vi "Flush Written TDMS Data.vi"() -> ()   [LabVIEW 2023]
doc: "Demonstrates the use of the TDMS Flush function to flush any written data from memory to the .tdms file on disk."
uses:
  <vilib>/Utility/TDMS File Viewer/NI_TDMS File Viewer.lvlib
panel:
  in  "Stop":bool
  out "Graph":waveform(dbl)[](graph)
  # "Overview: Demonstrates the use of the TDMS Flush function to flush any written data from memory to the .tdms file on disk.\nInstructions:\n1. Run this VI.\n2. Click the Stop button to stop this VI and view the data written to the .tdms file.\n3. Open the block diagram of this example to understand how to use the TDMS Flush function to ensure data integrity.\n4. Delete the .tdms file (located at [LabVIEW Data]\\Example Flush Written Data.tdms) when you are done."
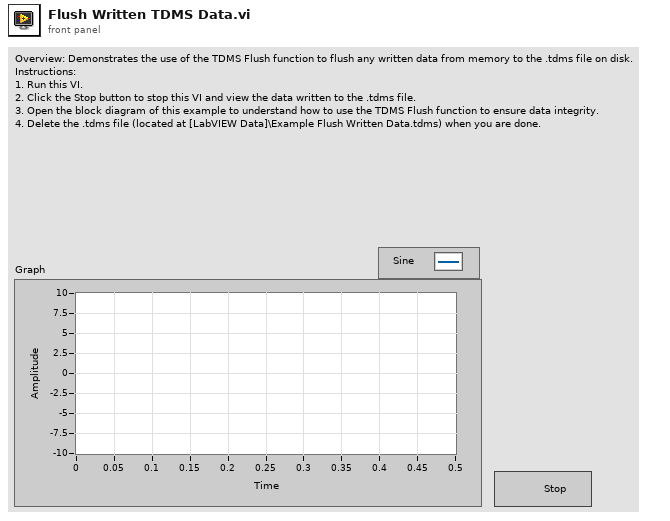
[diagram p1: front panel]
types:
  T1 = enum16{"open", "open or create", "create or replace", "create", "open (read-only)"}
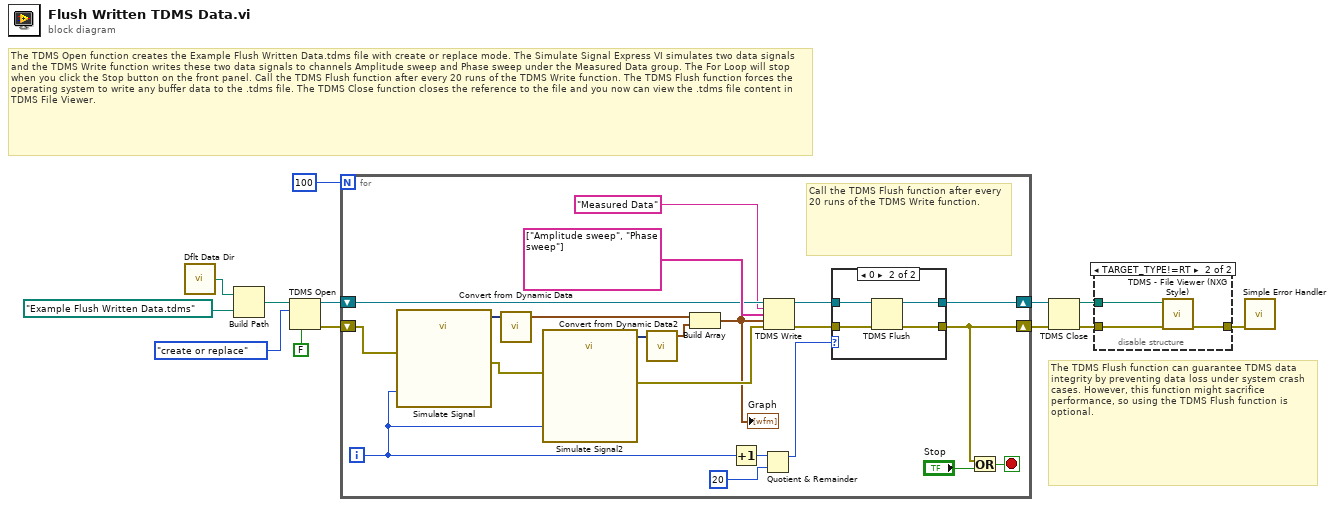
[diagram p0: block diagram]
diagram:
  # "The TDMS Flush function can guarantee TDMS data integrity by preventing data loss under system crash cases. However, this function might sacrifice performance, so using the TDMS Flush function is optional."
  # "The TDMS Open function creates the Example Flush Written Data.tdms file with create or replace mode. The Simulate Signal Express VI simulates two data signals and the TDMS Write function writes these two data signals to channels Amplitude sweep and Phase sweep under the Measured Data group. The For Loop will stop when you click the Stop button on the front panel. Call the TDMS Flush function after every 20 runs of the TDMS Write function. The TDMS Flush function forces the operating system to write any buffer data to the .tdms file. The TDMS Close function closes the reference to the file and you now can view the .tdms file content in TDMS File Viewer."
  n1 = call <vilib>:"Dflt Data Dir.vi"() -> ("App:Default Data Directory"=w13:path)
  n2 = Build Path(base path=w13, name or relative path=path "Example Flush Written Data.tdms" ("file path")) -> (appended path=w7:path)
  n3 = TDMS Open(6:FALSE ("disable buffering (T)"), 10:T1."create or replace" ("operation"), 11:w7) -> (0:w4:errorcluster, 3:w5:refnum<k34>)  [unwired: 4 in]
  n4 = for {
    N: 100 -> [_]
    shift-right: [w14] -> w2
    shift-left: w4 -> [w25]
    shift-right: [w16] -> w1
    shift-left: w5 -> [w24]
    i -> [w21]
    stop <- w23 stop-if-true
    # "Call the TDMS Flush function after every 20 runs of the TDMS Write function."
    n5 = call "Simulate Signal"("Amplitude"=w21, "error in (no error)"=w25) -> ("Sine"=w32:dynamicdata, "error out"=w31:errorcluster)  [unwired: 12 in]
    n6 = call "Convert from Dynamic Data"("Dynamic Data Type"=w32) -> ("Waveform"=w29:waveform(dbl))  [unwired: 3 in]
    n7 = call "Simulate Signal2"("Phase"=w21, "error in (no error)"=w31) -> ("Sine"=w30:dynamicdata, "error out"=w27:errorcluster)  [unwired: 12 in]
    n8 = call "Convert from Dynamic Data2"("Dynamic Data Type"=w30) -> ("Waveform"=w28:waveform(dbl))  [unwired: 3 in]
    n9 = Build Array(w29, w28) -> (w26:waveform(dbl)[])
    "Graph" <- w26
    n10 = Increment(x=w21) -> (x+1=w22:i32)
    n11 = Quotient & Remainder(x=w22, y=20) -> (x-y*floor(x/y)=w18:i32)  [unwired: 1 out]
    n12 = TDMS Write(0:w24, 5:"Measured Data", 7:string[] ["Amplitude sweep", "Phase sweep"] ("channel names"), 9:w26, 11:w27) -> (4:w17:refnum<k34>, 15:w19:errorcluster)  [unwired: 1 in, 2 out]
    n13 = case shown="0" w18 {
      tunnel: [w35 w40] -> w14
      tunnel: w19 -> [w35 w39]
      tunnel: w17 -> [w36 w38]
      tunnel: [w36 w37] -> w16
      frame Default {
      }
      frame 0 {
        n14 = TDMS Flush(4:w39, 7:w38) -> (0:w40:errorcluster, 3:w37:refnum<k34>)
      }
    }
    n15 = Or(x=w14, y="Stop") -> (x .or. y?=w23:bool)
  }
  n16 = TDMS Close(8:w2, 11:w1) -> (0:w11:errorcluster, 3:w9:path)
  n17 = disable-structure shown="TARGET_TYPE!=RT" {
    disable-tunnel: w11 -> [w41 w44]
    disable-tunnel: w9 -> [_ w43]
    disable-tunnel: [w41 w42] -> w8
    frame condition #0 {
    }
    frame condition #1 (active) {
      n18 = call <vilib>:"TDMS - File Viewer (NXG Style).vi"("error in"=w44, "file in"=w43) -> ("error out"=w42:errorcluster)  [unwired: 8 in, 1 out]
    }
  }
  n19 = call <vilib>:"Simple Error Handler.vi"("error in (no error)"=w8) -> ()  [unwired: 2 in, 7 out]
